vi "CSConnectGUI.contents.vi"() -> ()   [LabVIEW 2014, in "CSConnectGUI.lvlib"]
doc: "loads all VIs into memory - required for building an application"
uses:
  CSConnectGUI.lvlib
panel:
  out "error out":errorcluster
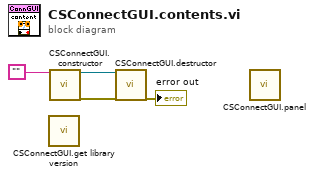
[diagram p0: block diagram]
diagram:
  n1 = call "CSConnectGUI.get library version.vi"() -> ()  [unwired: 1 in, 1 out]
  n2 = call "CSConnectGUI.constructor.vi"("name"="") -> ("i ref out"=w4:refnum<vi>, "error out"=w2:errorcluster)  [unwired: 16 in, 1 out]
  n3 = call "CSConnectGUI.destructor.vi"("i ref in"=w4, "error in (no error)"=w2) -> ("error out"=→"error out":errorcluster)  [unwired: 17 in]
  n4 = call "CSConnectGUI.panel.vi"() -> ()  [unwired: 12 in]
